vi "Send Reset Top Camera.vi"(8 "error in":errorcluster, 11 "Initialize to Default?":bool) -> (0 "error out":errorcluster)   [LabVIEW 2013]
uses:
  MsgQ Loops enum.ctl
  Main MsgQ.lvlib
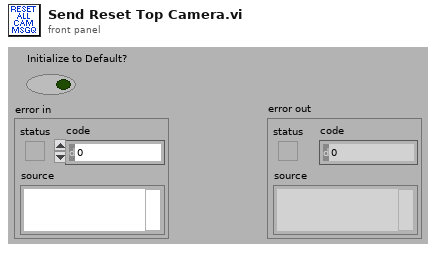
[diagram p1: front panel]
types:
  T1 = typedef "Main MsgQ.lvlib/MsgQ Loops enum.ctl" = enum16{"User Interface", "Image Acq"}
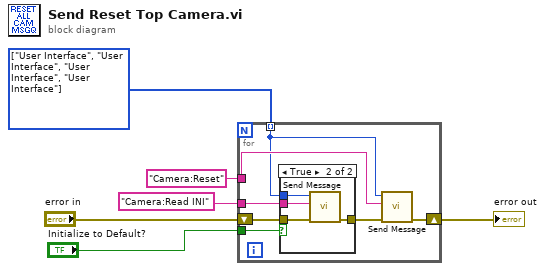
[diagram p0: block diagram]
diagram:
  w3 = T1[] [enum."User Interface", enum."User Interface", enum."User Interface", enum."User Interface"] items=["User Interface", "Image Acq"]
  n1 = for {
    tunnel: "Camera:Reset" ("Message String") -> [w13]
    tunnel: w3 -> [w9] mode=indexing
    shift-right: [w12] -> w4
    shift-left: "error in" -> [w11]
    tunnel: "Camera:Read INI" ("Message String") -> [w8]
    tunnel: "Initialize to Default?" -> [w7]
    n2 = case shown="True" w7 {
      tunnel: w11 -> [w14 w18]
      tunnel: [w14 w17] -> w10
      tunnel: w9 -> [_ w16]
      tunnel: w8 -> [_ w15]
      frame False {
      }
      frame True {
        n3 = call "Send Message.vi"("error in (no error)"=w18, "Message String"=w15, "Send to MsgQ"=w16) -> ("error out"=w17:errorcluster)  [unwired: 1 in, 7 out]
      }
    }
    n4 = call "Send Message.vi"("error in (no error)"=w10, "Message String"=w13, "Send to MsgQ"=w9) -> ("error out"=w12:errorcluster)  [unwired: 1 in, 7 out]
  }
  "error out" <- w4
